vi "Set Conditional Disable Value.vi"(8 "error in (no error)":errorcluster, 9 "Value":string, 10 "Key":string, 11 "Project Path":path) -> (0 "error out":errorcluster)   [LabVIEW 2024]
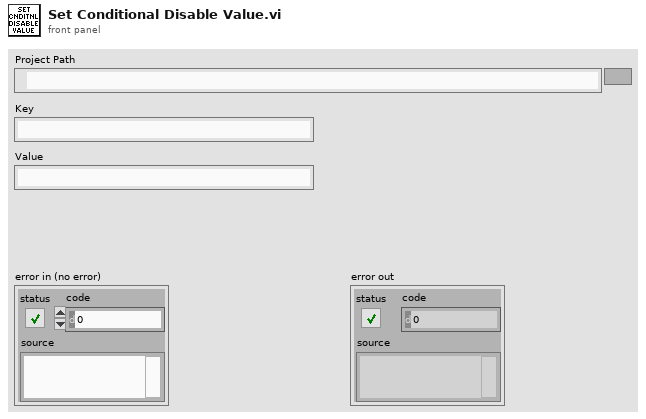
[diagram p1: front panel]
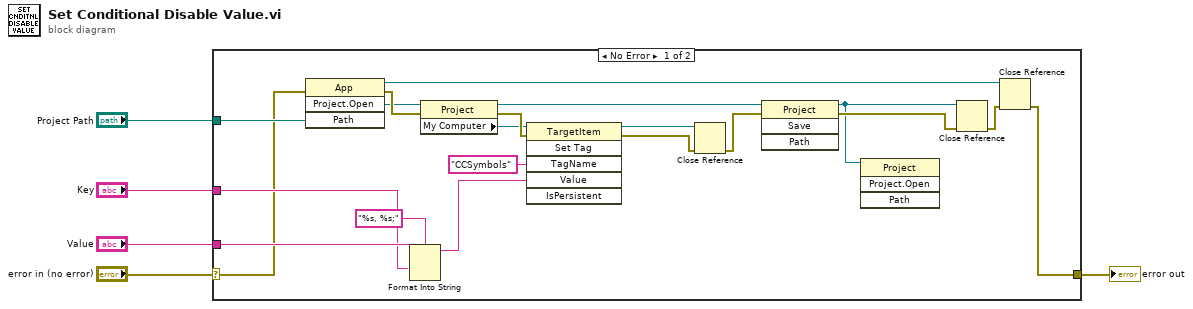
[diagram p0: block diagram]
diagram:
  n1 = case shown="No Error" "error in (no error)" {
    selector: "error in (no error)" -> [w7 w26]
    tunnel: [w25 w26] -> w5
    tunnel: "Value" -> [w15 _]
    tunnel: "Key" -> [w14 _]
    tunnel: "Project Path" -> [w8 _]
    frame No Error {
      n2 = invoke class="App" method="Project.Open"(error in=w7, "Path"=w8) -> (reference out=w23:refnum<vi>, error out=w10:errorcluster, "Project:Open"=w9:refnum<vi>)  [unwired: 2 in, 1 out]
      n3 = Format Into String(format string="%s, %s;", w14, w15) -> (resulting string=w16:string)  [unwired: 2 in, 1 out]
      n4 = property class="Project"(reference=w9, error in=w10) -> (reference out=w18:refnum<vi>, error out=w21:errorcluster, "My Computer"=w11:refnum<vi>)
      n5 = invoke class="TargetItem" method="Set Tag"(reference=w11, error in=w21, "TagName"="CCSymbols" ("Tag Name"), "Value"=w16) -> (reference out=w17:refnum<vi>, error out=w20:errorcluster)  [unwired: 2 in, 4 out]
      n6 = Close Reference(reference=w17, error in (no error)=w20) -> (error out=w19:errorcluster)
      n7 = invoke class="Project" method="Save"(reference=w18, error in=w19) -> (reference out=w6:refnum<vi>, error out=w22:errorcluster)  [unwired: 2 in, 2 out]
      n8 = invoke class="Project" method="Project.Open"(reference=w6) -> ()  [unwired: 3 in, 4 out]
      n9 = Close Reference(reference=w6, error in (no error)=w22) -> (error out=w24:errorcluster)
      n10 = Close Reference(reference=w23, error in (no error)=w24) -> (error out=w25:errorcluster)
    }
    frame Error {
    }
  }
  "error out" <- w5
